vi "Configure OPP.vi"(0 "VISA resource name":refnum<visa-resource-name>, 5 "Power Limit (150.00 W)":dbl=150.0 min=0.0 max=6050.0 step=0.01 format="%.2g", 7 "Protection Delay (0)":dbl min=0.0 max=60.0 step=1.0 format="%#.3f", 9 "Hardware Power Limit (150 W)":dbl=150.0 min=0.0 max=6000.0 step=1.0, 11 "error in (no error)":errorcluster) -> (4 "VISA resource name out":refnum<visa-resource-name>, 15 "error out":errorcluster)   [LabVIEW 2018, in "BK Precision 8600 Series.lvlib"]
doc: "Configures over power protection (OPP) and the hardware power protection limit."
uses:
  <instrlib>/BK Precision 8600 Series/BK Precision 8600 Series.lvlib
panel:
  # "W"
  # "s"
  # "W"
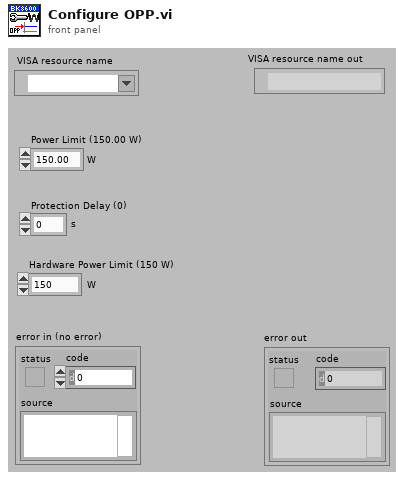
[diagram p1: front panel]
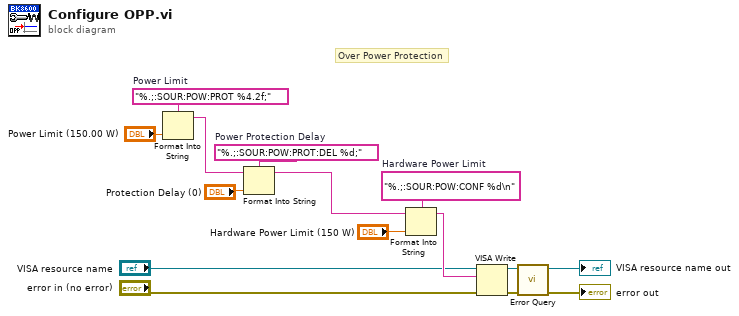
[diagram p0: block diagram]
diagram:
  w9 = "%.;:SOUR:POW:CONF %d\n"  # Hardware Power Limit
  w14 = "%.;:SOUR:POW:PROT:DEL %d;"  # Power Protection Delay
  w15 = "%.;:SOUR:POW:PROT %4.2f;"  # Power Limit
  # "Over Power Protection"
  n1 = Format Into String(format string=w15, "Power Limit (150.00 W)") -> (resulting string=w13:string)  [unwired: 2 in, 1 out]
  n2 = Format Into String(format string=w14, initial string=w13, "Protection Delay (0)") -> (resulting string=w8:string)  [unwired: 1 in, 1 out]
  n3 = Format Into String(format string=w9, initial string=w8, "Hardware Power Limit (150 W)") -> (resulting string=w7:string)  [unwired: 1 in, 1 out]
  n4 = VISA Write(VISA resource name="VISA resource name", write buffer=w7, error in (no error)="error in (no error)") -> (VISA resource name out=w6:refnum<visa-resource-name>, error out=w5:errorcluster)  [unwired: 1 out]
  n5 = call <instrlib>:"Error Query.vi"("error in (no error)"=w5, "VISA resource name"=w6) -> ("error out"=→"error out":errorcluster, "VISA resource name out"=→"VISA resource name out":refnum<visa-resource-name>)  [unwired: 6 in, 2 out]
